vi "next.vi"() -> ()   [LabVIEW 2019]
uses:
  <vilib>/userDefined/High Color/IMAQdx.ctl
  <vilib>/vision/driver/NI_Vision_Acquisition_Software.lvlib
panel:
  out "Image":T1(plugin-control)
  in  "stop":bool
  out "Image 2":T1(plugin-control)
  out "String (OCR/OCV 1)":string
  in  "File Path (OCR/OCV 1)":path=path "D:/3下課程/總結式課程/影像/OCR/train1.abc"
  in  "Rectangle":T2 {"Rotation" min=-90.0 max=90.0 step=1.0 format="%.2f"; "Left" scale=0.0..1024.0; "Right" scale=0.0..1024.0}
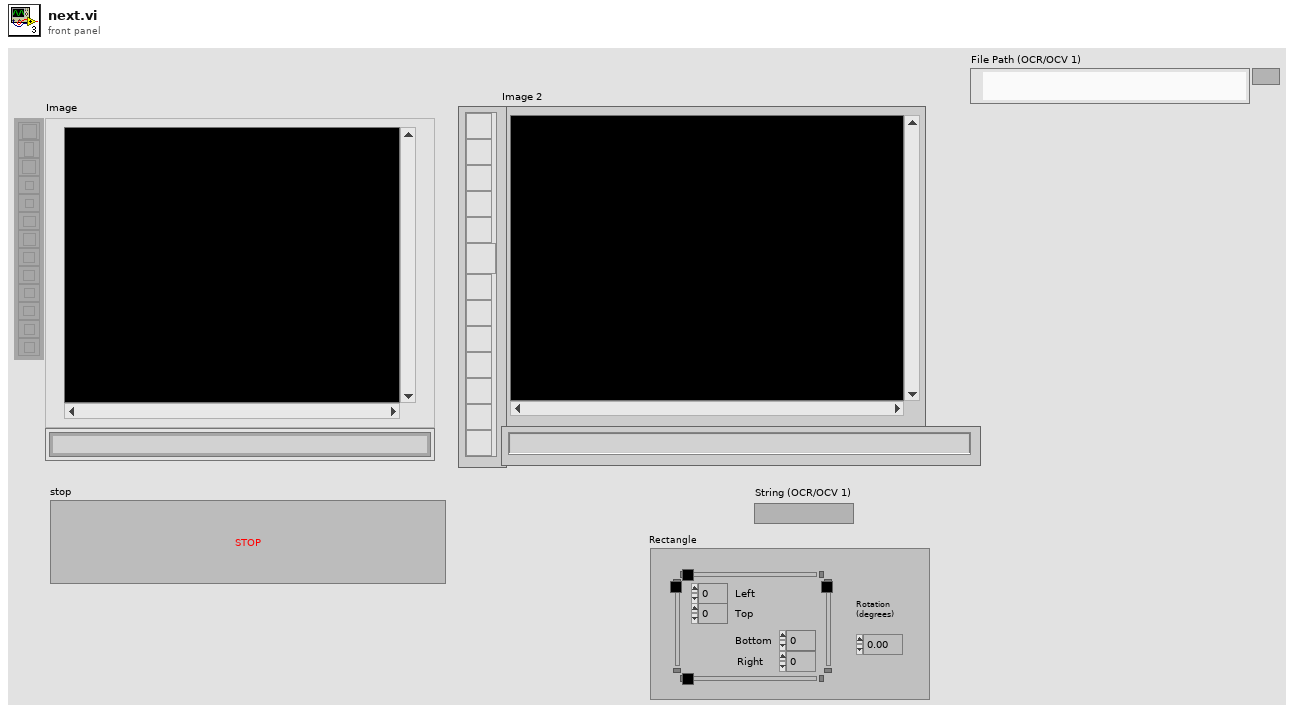
[diagram p1: front panel]
types:
  T1 = typedef "IMAQ Image.ctl" = refnum<image>
  T2 = typedef "IMAQ Rectangle" = cluster{"Left":i32, "Top":i32, "Right":i32, "Bottom":i32, "Rotation":dbl}
  T3 = typedef "Image Type" = u32
  T4 = typedef "IMAQdx.ctl" = refnum<k21>
  T5 = typedef "ROI Descriptor" = cluster{"Global Rectangle":i32[], "Contours":cluster{"ID":enum32{"External", "Internal"}, "Type":u32, "Coordinates":i32[]}[]}
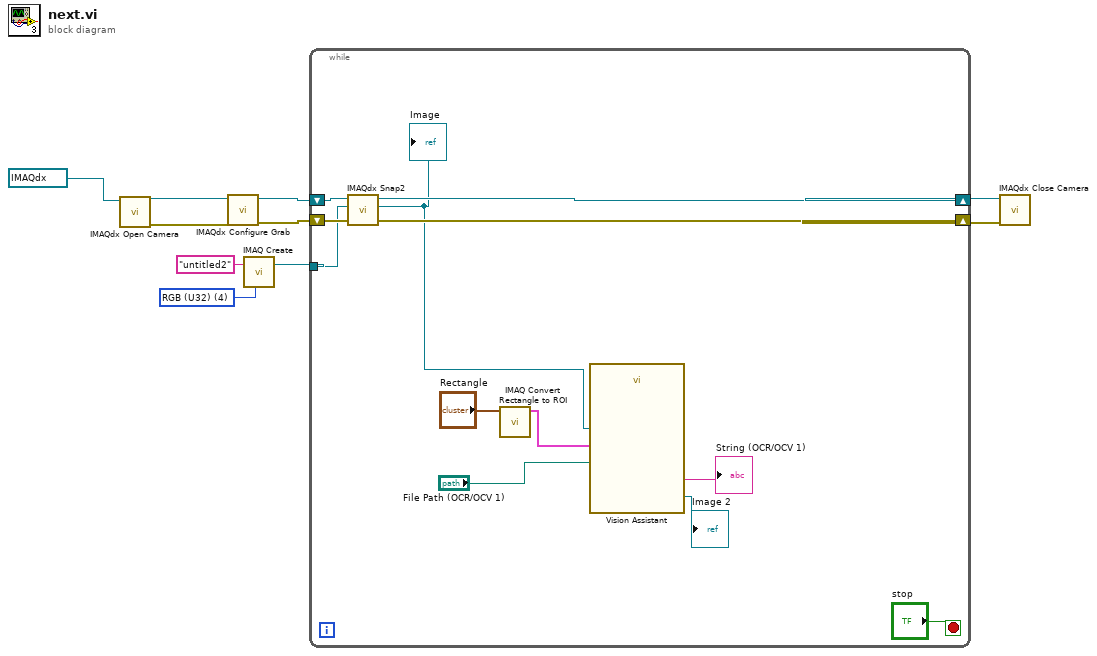
[diagram p0: block diagram]
diagram:
  w1 = T3 4 items=["Grayscale (U8)", "Grayscale (I16)", "Grayscale (SGL)", "Complex (CSG)", "RGB (U32)", "HSL (U32)", "RGB (U64)", "Grayscale (U16)"] ("Image Type")
  n1 = call <vilib>:"IMAQdx Open Camera.vi"("Session In"=T4 "cam1") -> ("error out"=w6:errorcluster, "Session Out"=w9:T4)  [unwired: 9 in]
  n2 = call <vilib>:"IMAQdx Configure Grab.vi"("error in"=w6, "Session In"=w9) -> ("error out"=w5:errorcluster, "Session Out"=w8:T4)  [unwired: 8 in]
  n3 = call "IMAQ Create"("Image Name"="untitled2", "Image Type"=w1) -> ("New Image"=w2:T1)  [unwired: 3 in, 1 out]
  n4 = while {
    tunnel: w2 -> [w16]
    shift-right: [w21] -> w7
    shift-left: w8 -> [w22]
    shift-right: [w19] -> w4
    shift-left: w5 -> [w20]
    stop <- "stop" stop-if-true
    n5 = call <vilib>:"IMAQdx Snap2.vi"("error in"=w20, "Image In"=w16, "Session In"=w22) -> ("error out"=w19:errorcluster, "Image Out"=w11:T1, "Session Out"=w21:T4)  [unwired: 6 in]
    "Image" <- w11
    n6 = call "IMAQ Convert Rectangle to ROI"("Rectangle"="Rectangle") -> ("ROI Descriptor"=w12:T5)  [unwired: 8 in, 1 out]
    n7 = call "Vision Assistant"("Image In"=w11, "ROI Descriptor (OCR/OCV 1)"=w12, "File Path (OCR/OCV 1)"="File Path (OCR/OCV 1)") -> ("Image Out"=→"Image 2":T1, "String (OCR/OCV 1)"=→"String (OCR/OCV 1)":string)  [unwired: 22 in, 1 out]
  }
  n8 = call <vilib>:"IMAQdx Close Camera.vi"("error in"=w4, "Session In"=w7) -> ()  [unwired: 9 in, 1 out]
